vi "hamamatsuClose.vi"() -> (0 "error out":errorcluster {"code" format="%.0x"})   [LabVIEW 2017]
uses:
  globalDevices.vi
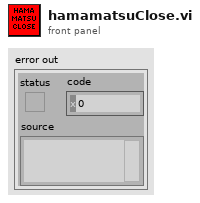
[diagram p1: front panel]
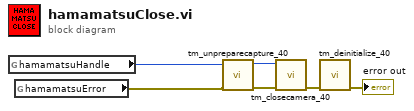
[diagram p0: block diagram]
diagram:
  n1 = global read "globalDevices.vi" "hamamatsuHandle"() -> (w2:u32)
  n2 = global read "globalDevices.vi" "hamamatsuError"() -> (w1:errorcluster)
  n3 = call <userlib>:"tm_unpreparecapture_40.vi"("error in (no error)"=w1, "Handle in"=w2) -> ("error out"=w6:errorcluster, "Handle out"=w5:u32)  [unwired: 8 in]
  n4 = call <userlib>:"tm_closecamera_40.vi"("error in (no error)"=w6, "Handle in"=w5) -> ("error out"=w4:errorcluster)  [unwired: 9 in]
  n5 = call <userlib>:"tm_deinitialize_40.vi"("error in (no error)"=w4) -> ("error out"=→"error out":errorcluster)  [unwired: 10 in]
